vi "PUT Z Scan Size [Slope Calibration].vi"(0 "Z Scan Size":dbl) -> ()   [LabVIEW 2013]
uses:
  Action.ctl
  Slope Calibration Inputs FGV Selector.ctl
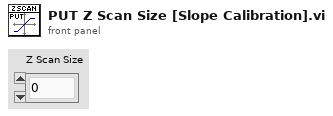
[diagram p1: front panel]
types:
  T1 = typedef "Slope Calibration Inputs FGV Selector.ctl" = enum16{"Number of Samples", "Ramp Rate", "Z Scan Size"}
  T2 = typedef "Action.ctl" = enum16{"GET", "PUT", "DELETE"}
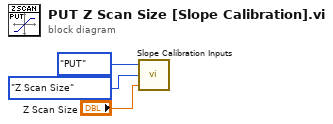
[diagram p0: block diagram]
diagram:
  n1 = call "Slope Calibration Inputs.vi"("Input"="Z Scan Size", "Slope Calibration Inputs FGV Selector"=Slope_Calibration_Inputs_FGV_Selector."Z Scan Size", "Action"=Action."PUT") -> ()  [unwired: 1 out]
